vi "GetNameOfSampleCalFile.vi"(8 "Error In":errorcluster, 11 "Position":i16) -> (0 "Error Out":errorcluster, 3 "Filename":string)   [LabVIEW 2019]
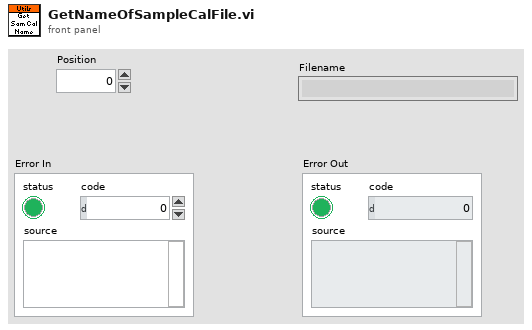
[diagram p1: front panel]
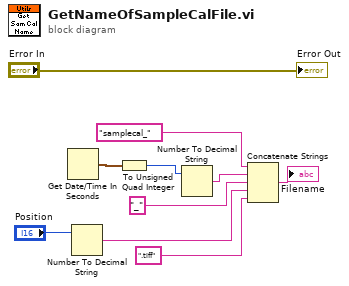
[diagram p0: block diagram]
diagram:
  n1 = Get Date/Time In Seconds() -> (seconds since 1Jan1904=w10:timestamp)
  n2 = Number To Decimal String(number="Position") -> (decimal integer string=w1:string)  [unwired: 1 in]
  n3 = To Unsigned Quad Integer(1:w10) -> (0:w9:u64)
  n4 = Number To Decimal String(number=w9) -> (decimal integer string=w7:string)  [unwired: 1 in]
  n5 = Concatenate Strings("samplecal_", w7, "_" ("string"), w1, ".tiff" ("string")) -> (→"Filename":string)
  "Error Out" <- "Error In"
